vi "test_GetItemInformationFromProjects_SampleVilibProject.vi"() -> (3 "Pass?":bool)   [LabVIEW 2019, in "Tests.SolutionBuilder.lvlib"]
uses:
  Tests.SolutionBuilder.lvlib
  SolutionBuilder/SolutionBuilder.lvclass
  SolutionBuilder/ProjectItem/ProjectItem.lvclass
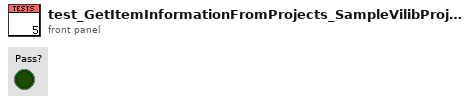
[diagram p1: front panel]
types:
  T1 = typedef "SolutionBuilder.lvlib/SolutionBuilder.lvclass/ProjectItemMap.ctl" = map{path, refnum<class "ProjectItem.lvclass">[]}
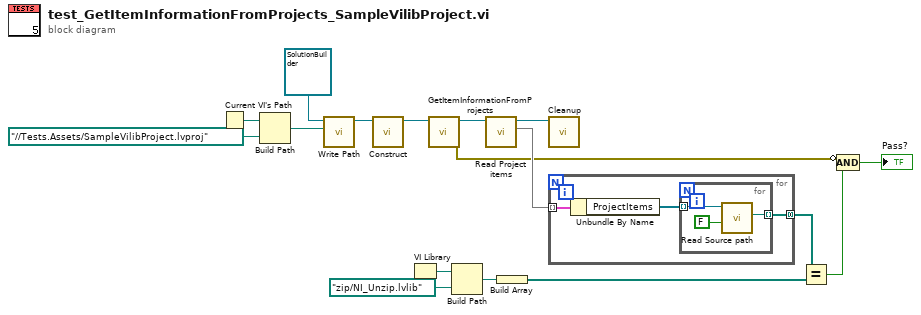
[diagram p0: block diagram]
diagram:
  n1 = Current VI's Path() -> (path=w16:path)
  n2 = Build Path(base path=w16, name or relative path=path "../../Tests.Assets/SampleVilibProject.lvproj" ("Path")) -> (appended path=w14:path)
  n3 = call "Write Path.vi"("Path"=w14, "SolutionBuilder in"=refnum<class "SolutionBuilder.lvclass"> refnum) -> ("SolutionBuilder out"=w12:refnum<class "SolutionBuilder.lvclass">)  [unwired: 9 in]
  n4 = call "Construct.vi"("SolutionBuilder in"=w12) -> ("SolutionBuilder out"=w8:refnum<class "SolutionBuilder.lvclass">)  [unwired: 9 in, 1 out]
  n5 = VI Library() -> (path=w4:path)
  n6 = call "GetItemInformationFromProjects.vi"("SolutionBuilder in"=w8) -> ("error out"=w6:errorcluster, "SolutionBuilder out"=w7:refnum<class "SolutionBuilder.lvclass">)  [unwired: 9 in]
  n7 = Build Path(base path=w4, name or relative path=path "zip/NI_Unzip.lvlib" ("Path")) -> (appended path=w3:path)
  n8 = call "Read Project items.vi"("SolutionBuilder in"=w7) -> ("Project items"=w13:T1, "SolutionBuilder out"=w10:refnum<class "SolutionBuilder.lvclass">)  [unwired: 9 in]
  n9 = Build Array(w3) -> (w2:path[])
  n10 = call "Cleanup.vi"("SolutionBuilder in"=w10) -> ()  [unwired: 9 in, 2 out]
  n11 = for {
    tunnel: w13 -> [w20] mode=indexing
    tunnel: [w18] -> w9 mode=concatenating
    n12 = Unbundle By Name(w20) -> ("ProjectItems"=w19:refnum<class "ProjectItem.lvclass">[])
    n13 = for {
      tunnel: w19 -> [w23] mode=indexing
      tunnel: [w21] -> w18 mode=indexing
      n14 = call "Read Source path.vi"("Force abs path? (T)"=FALSE, "ProjectItem in"=w23) -> ("Source path"=w21:path)  [unwired: 8 in, 1 out]
    }
  }
  n15 = Equal?(x=w9, y=w2) -> (x = y?=w11:bool)
  n16 = Compound Arithmetic op=AND(invert w6, w11) -> (→"Pass?":bool)
